vi "Initialize_Position Save Module.vi"(8 "Error In":errorcluster, 11 "UI Controls Refnum":T1) -> (0 "Error Out":errorcluster)   [LabVIEW 2012]
uses:
  Custom Control and Typedefs/UI Controls Refnum.ctl
  Custom Control and Typedefs/ChannelSelector_for_PosSave.ctl
  Custom Controls/PositionSaveMod.ctl
  Custom Control and Typedefs/Overlay Control.ctl
  CommonResource VIs/UI Control and Indicator properties_Commands.ctl
  PositionSaveFGVCommands.ctl
  CommonResource VIs/FormatTableStyle_Commands.ctl
  Image Validity FGV_Commands.ctl
  Custom Controls/MAIN Image panel tab Control type def.ctl
  Custom Controls/MAIN Image panel reso tab Control type def.ctl
  Chnl_2_tab_Commands.ctl
  GFG/GFG library.lvlib
panel:
  # "Red (Current Image)"
  # "Green (Saved Image)"
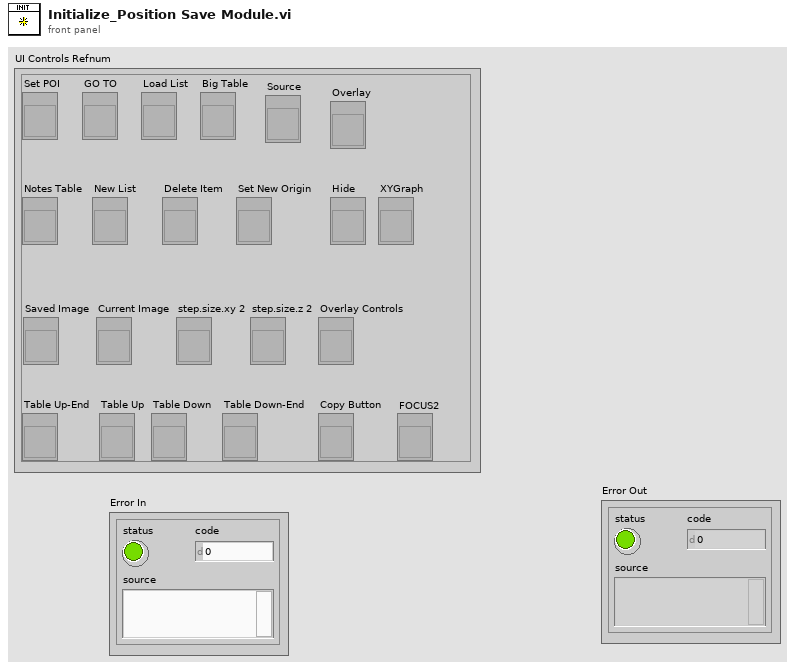
[diagram p1: front panel]
types:
  T1 = typedef "UI Controls Refnum.ctl" = cluster{"GO TO":refnum<vi>, "Load List":refnum<vi>, "Big Table":refnum<vi>, "Notes Table":refnum<vi>, "New List":refnum<vi>, "Delete Item":refnum<vi>, "Set New Origin":refnum<vi>, "Set POI":refnum<vi>, "Saved Image":refnum<vi>, "Current Image":refnum<vi>, "step.size.xy 2":refnum<vi>, "step.size.z 2":refnum<vi>, "Source":refnum<vi>, "Table Up-End":refnum<vi>, "Table Up":refnum<vi>, "Table Down":refnum<vi>, "Table Down-End":refnum<vi>, "Copy Button":refnum<vi>, "Hide":refnum<vi>, "Overlay Controls":refnum<vi>, "Overlay":refnum<vi>, "XYGraph":refnum<vi>, "FOCUS2":refnum<vi>}
  T2 = typedef "PositionSaveMod.ctl" = bool
  T3 = typedef "Image Validity FGV_Commands.ctl" = enum16{"Set validity status", "Get Validity status"}
  T4 = typedef "FormatTableStyle_Commands.ctl" = enum16{"Colour Row", "Uncolour Row", "Bold Row", "Clear table", "UpdateVisibleRows"}
  T5 = typedef "PositionSaveFGVCommands.ctl" = enum16{"Initialize", "NewList", "LoadList", "CopyList", "DeleteSelected", "SetPosition", "SetNewOrigin", "UpdateEntireTable", "GetPosition", "Shutdown and Cleanup"}
  T6 = typedef "UI Control and Indicator properties_Commands.ctl" = enum16{"Enable", "Disable", "Disable and Grey", "Make Visible", "Make Invisible"}
  T7 = typedef "Chnl_2_tab_Commands.ctl" = enum16{"ChannelToTab", "TabToChannel"}
  T8 = typedef "MAIN Image panel reso tab Control type def.ctl" = enum32{"Channel 1", "Channel 2", "Channel 3", "Channel 4", "Channel 5", "all channels", "RGB overlay", "ROI", "arbitrary line scan"}
  T9 = typedef "MAIN Image panel tab Control type def.ctl" = enum32{"Channel 1", "Channel 2", "Channel 3", "Channel 4", "all channels", "RGB overlay", "ROI", "arbitrary line scan"}
  T10 = typedef "ChannelSelector_for_PosSave.ctl" = enum16{"Channel 1", "Channel 2", "Channel 3", "Channel 4"}
  T11 = cluster{"WaveformChartRef":refnum<vi>, "DigitalRef":refnum<vi>, "ArrayRef":refnum<vi>, "TabControlRef":refnum<vi>, "EnumRef":refnum<vi>, "RingRef":refnum<vi>, "BooleanRef":refnum<vi>, "KnobRef":refnum<vi>, "SlideRef":refnum<vi>, "PathRef":refnum<vi>, "StringRef":refnum<vi>, "ComboBox":refnum<vi>, "WaveformGraphRef":refnum<vi>}
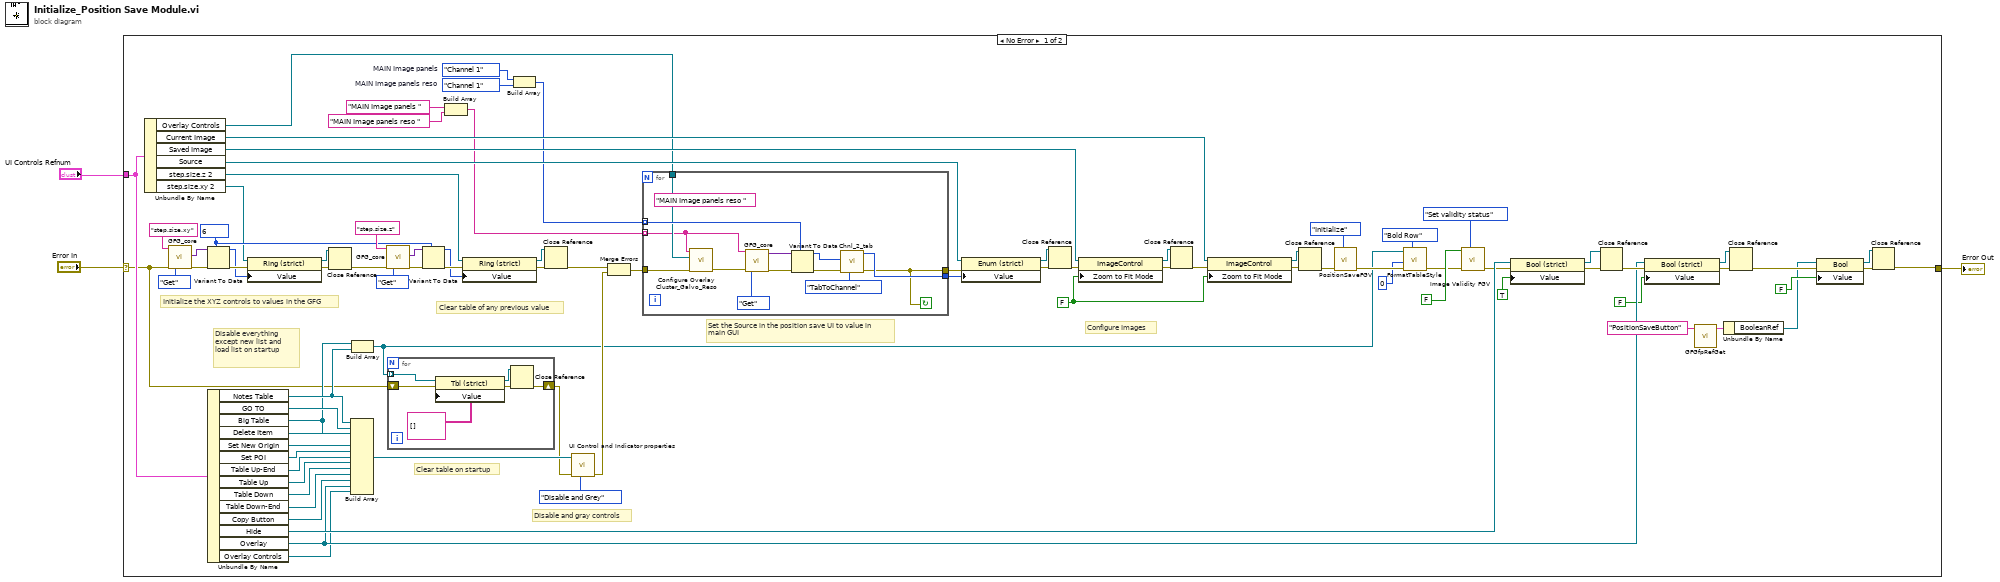
[diagram p0: block diagram]
diagram:
  n1 = case shown="No Error" "Error In" {
    selector: "Error In" -> [w48 w111]
    tunnel: "UI Controls Refnum" -> [w51 _]
    tunnel: [w5 w111] -> w1
    frame No Error {
      w14 = MAIN_Image_panel_reso_tab_Control_type_def."Channel 1"  # MAIN Image panels reso
      w15 = MAIN_Image_panel_tab_Control_type_def."Channel 1"  # MAIN Image panels
      w73 = FALSE ("Zoom to Fit Mode")
      w81 = u16 6 items=["  1"=1, "  2"=2, "  5"=5, " 10"=10, " 20"=20, " 50"=50, "100"=100] ("step.size.xy 2")
      # "Disable and gray controls"
      # "Clear table on startup"
      # "Clear table of any previous value"
      # "Disable everything except new list and load list on startup"
      # "Configure Images"
      # "Set the Source in the position save UI to value in \nmain GUI"
      # "Initialize the XYZ controls to values in the GFG"
      n2 = Unbundle By Name(w51) -> ("Overlay Controls"=w4:refnum<vi>, "Current Image"=w63:refnum<vi>, "Saved Image"=w64:refnum<vi>, "Source"=w74:refnum<vi>, "step.size.z 2"=w76:refnum<vi>, "step.size.xy 2"=w77:refnum<vi>)
      n3 = call "GFG_core.vi"("Variable Name in"="step.size.xy", "error in (no error)"=w48, "Action"=enum16{"Init", "Set", "Get"}."Get") -> ("Variant Out"=w86:variant, "error out"=w87:errorcluster)  [unwired: 10 in, 5 out]
      n4 = Variant To Data(error in=w87, type=w81, Variant=w86) -> (data=w84:u16, error out=w85:errorcluster)
      n5 = Unbundle By Name(w51) -> ("Notes Table"=w50:refnum<vi>, "GO TO"=w57:refnum<vi>, "Big Table"=w49:refnum<vi>, "Delete Item"=w56:refnum<vi>, "Set New Origin"=w55:refnum<vi>, "Set POI"=w54:refnum<vi>, "Table Up-End"=w41:refnum<vi>, "Table Up"=w40:refnum<vi>, "Table Down"=w39:refnum<vi>, "Table Down-End"=w38:refnum<vi>, "Copy Button"=w27:refnum<vi>, "Hide"=w26:refnum<vi>, "Overlay"=w20:refnum<vi>, "Overlay Controls"=w16:refnum<vi>)
      n6 = property on="Property Node" class="Ring (strict)"(reference=w77, error in=w85, "Value"=w84) -> (reference out=w71:refnum<vi>, error out=w72:errorcluster)
      n7 = Close Reference(reference=w71, error in (no error)=w72) -> (error out=w70:errorcluster)
      n8 = Build Array(w50, w57, w49, w56, w55, w54, w41, w40, w39, w38, w27, w20, w16) -> (w53:refnum<vi>[])
      n9 = Build Array(w49, w50) -> (w34:refnum<vi>[])
      n10 = call "GFG_core.vi"("Variable Name in"="step.size.z", "error in (no error)"=w70, "Action"=enum16{"Init", "Set", "Get"}."Get") -> ("Variant Out"=w82:variant, "error out"=w83:errorcluster)  [unwired: 10 in, 5 out]
      n11 = for {
        tunnel: w34 -> [w109] mode=indexing
        shift-right: [w105] -> w47
        shift-left: w48 -> [w108]
        n12 = property class="Tbl (strict)"(reference=w109, error in=w108, "Value"=string[][] []) -> (reference out=w106:refnum<vi>, error out=w107:errorcluster)
        n13 = Close Reference(reference=w106, error in (no error)=w107) -> (error out=w105:errorcluster)
      }
      n14 = Variant To Data(error in=w83, type=w81, Variant=w82) -> (data=w79:u16, error out=w80:errorcluster)
      n15 = Build Array("MAIN Image panels " ("Variable Name in"), "MAIN Image panels reso " ("Variable Name in")) -> (w31:string[])
      n16 = property on="Property Node" class="Ring (strict)"(reference=w76, error in=w80, "Value"=w79) -> (reference out=w68:refnum<vi>, error out=w69:errorcluster)
      n17 = Build Array(w15, w14) -> (w13:u32[])
      n18 = Close Reference(reference=w68, error in (no error)=w69) -> (error out=w45:errorcluster)
      n19 = call "UI Control and Indicator properties.vi"("Enable Command"=UI_Control_and_Indicator_properties_Commands."Disable and Grey", "Error In"=w47, "Control Refnums"=w53) -> ("Error Out"=w44:errorcluster)  [unwired: 8 in]
      n20 = Merge Errors(w45, w44) -> (w46:errorcluster)
      n21 = for {
        tunnel: [w102] -> w78
        tunnel: [w96] -> w75
        tunnel: w46 -> [w95]
        tunnel: w31 -> [w92] mode=indexing
        tunnel: w13 -> [w97] mode=indexing
        tunnel: w4 -> [w93]
        stop <- w96 continue-if-true
        (unwired) "MAIN Image panels reso " ("Variable Name in")
        n22 = call "Configure Overlay Cluster_Galvo_Reso.vi"("Error In"=w95, "Overlay Control Reference"=w93, "Overlay Control Type"=w92) -> ("Error Out"=w94:errorcluster)  [unwired: 8 in]
        n23 = call "GFG_core.vi"("Variable Name in"=w92, "error in (no error)"=w94, "Action"=enum16{"Init", "Set", "Get"}."Get") -> ("Variant Out"=w104:variant, "error out"=w103:errorcluster)  [unwired: 10 in, 5 out]
        n24 = Variant To Data(error in=w103, type=w97, Variant=w104) -> (data=w98:u32, error out=w100:errorcluster)
        n25 = call "Chnl_2_tab.vi"("Command"=Chnl_2_tab_Commands."TabToChannel", "Error In"=w100, "Tab IN"=w98) -> ("Error Out"=w96:errorcluster, "Channel  OUT"=w102:T10)  [unwired: 6 in, 1 out]
      }
      n26 = property on="Property Node" class="Enum (strict)"(reference=w74, error in=w75, "Value"=w78) -> (reference out=w66:refnum<vi>, error out=w67:errorcluster)
      n27 = Close Reference(reference=w66, error in (no error)=w67) -> (error out=w65:errorcluster)
      n28 = property class="ImageControl"(reference=w64, error in=w65, "Zoom to Fit Mode"=w73) -> (reference out=w61:refnum<vi>, error out=w62:errorcluster)
      n29 = Close Reference(reference=w61, error in (no error)=w62) -> (error out=w58:errorcluster)
      n30 = property class="ImageControl"(reference=w63, error in=w58, "Zoom to Fit Mode"=w73) -> (reference out=w59:refnum<vi>, error out=w60:errorcluster)
      n31 = Close Reference(reference=w59, error in (no error)=w60) -> (error out=w43:errorcluster)
      n32 = call "PositionSaveFGV.vi"("PositionSave Commands"=PositionSaveFGVCommands."Initialize", "Error In"=w43) -> ("Error Out"=w37:errorcluster)  [unwired: 5 in, 4 out]
      n33 = call "FormatTableStyle.vi"("Format Command"=FormatTableStyle_Commands."Bold Row", "Error In"=w37, "Row Index"=0 ("Row"), "Table reference Array"=w34) -> ("Error Out"=w28:errorcluster)  [unwired: 7 in]
      n34 = call "Image Validity FGV.vi"("Image Validity FGV_Commands"=Image_Validity_FGV_Commands."Set validity status", "Error In"=w28, "Validity status IN"=FALSE) -> ("Error Out"=w24:errorcluster)  [unwired: 7 in, 1 out]
      n35 = property class="Bool (strict)"(reference=w26, error in=w24, "Value"=T2 TRUE) -> (reference out=w22:refnum<vi>, error out=w23:errorcluster)
      n36 = Close Reference(reference=w22, error in (no error)=w23) -> (error out=w21:errorcluster)
      n37 = property class="Bool (strict)"(reference=w20, error in=w21, "Value"=FALSE) -> (reference out=w17:refnum<vi>, error out=w19:errorcluster)
      n38 = call "GFGfpRefGet.vi"("Variable Name in"="PositionSaveButton") -> ("output cluster"=w11:T11)  [unwired: 9 in, 1 out]
      n39 = Unbundle By Name(w11) -> ("BooleanRef"=w8:refnum<vi>)
      n40 = Close Reference(reference=w17, error in (no error)=w19) -> (error out=w10:errorcluster)
      n41 = property class="Bool"(reference=w8, error in=w10, "Value"=FALSE) -> (reference out=w6:refnum<vi>, error out=w7:errorcluster)
      n42 = Close Reference(reference=w6, error in (no error)=w7) -> (error out=w5:errorcluster)
    }
    frame Error {
    }
  }
  "Error Out" <- w1
